vi "medicaoIXV.vi"() -> ()   [LabVIEW 2012]
uses:
  <vilib>/Utility/file.llb/Write To Spreadsheet File (string).vi
  <vilib>/Utility/file.llb/Write To Spreadsheet File (DBL).vi
  <instrlib>/Agilent 6XXX Series/Agilent 6XXX Series.lvlib
panel:
  out "PmpTemp":dbl
  out "stop2":bool
  out "reset graph":bool=TRUE
  out "array":dbl[][](array[numeric])
  in  "Tab Control":enum32{"Entrada de dados", "Saída de dados"}(tab)
  in  "Formato":u16(ring) items=[".txt", ".csv"]
  out "ON/OFF":bool
  in  "Pontos":dbl
  in  "Tensão máxima":dbl
  in  "Nome da célula":string
  in  "Local":path
  in  "Delay(ms)":dbl
  in  "Start":bool
  out "Icc (A)":dbl
  out "Vca (V)":dbl
  in  "Print Screen":bool
  out "IXV":cluster{"Y":dbl[], "Y":dbl[]}[](graph)
  out "output voltage":dbl
  out "Tensao Atual (V)":dbl
  out "Corrente Atual\n(A)":dbl
  out "Ponto Atual":i32
  out "TABELA DE DADOS\nTensão(fonte)     Tensão                  Corrente            Pontos":dbl[][](array[numeric]) caption="all rows" format="%0.3f"
  in  "stop":bool
  out "ON/OFF":bool
  in  "CorrenteGraph":dbl
  in  "error in (no error)":errorcluster
  out "error out":errorcluster
  in  "TensaoGraph":dbl
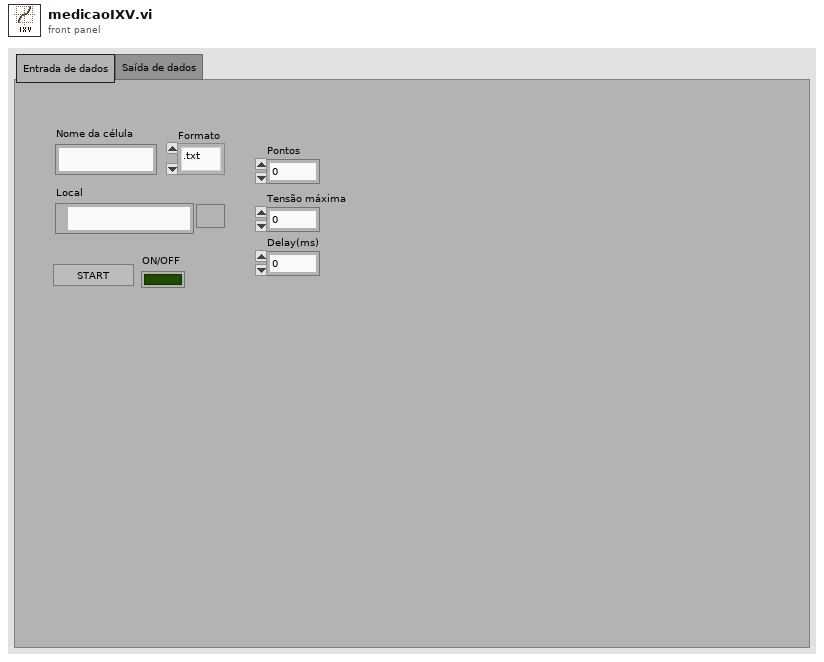
[diagram p1: front panel]
types:
  T1 = typedef "imagedata.ctl" = cluster{"image type":i32, "image depth":i32, "image":u8[], "mask":u8[], "colors":u32[], "Rectangle":cluster{"left":i16, "top":i16, "right":i16, "bottom":i16}}
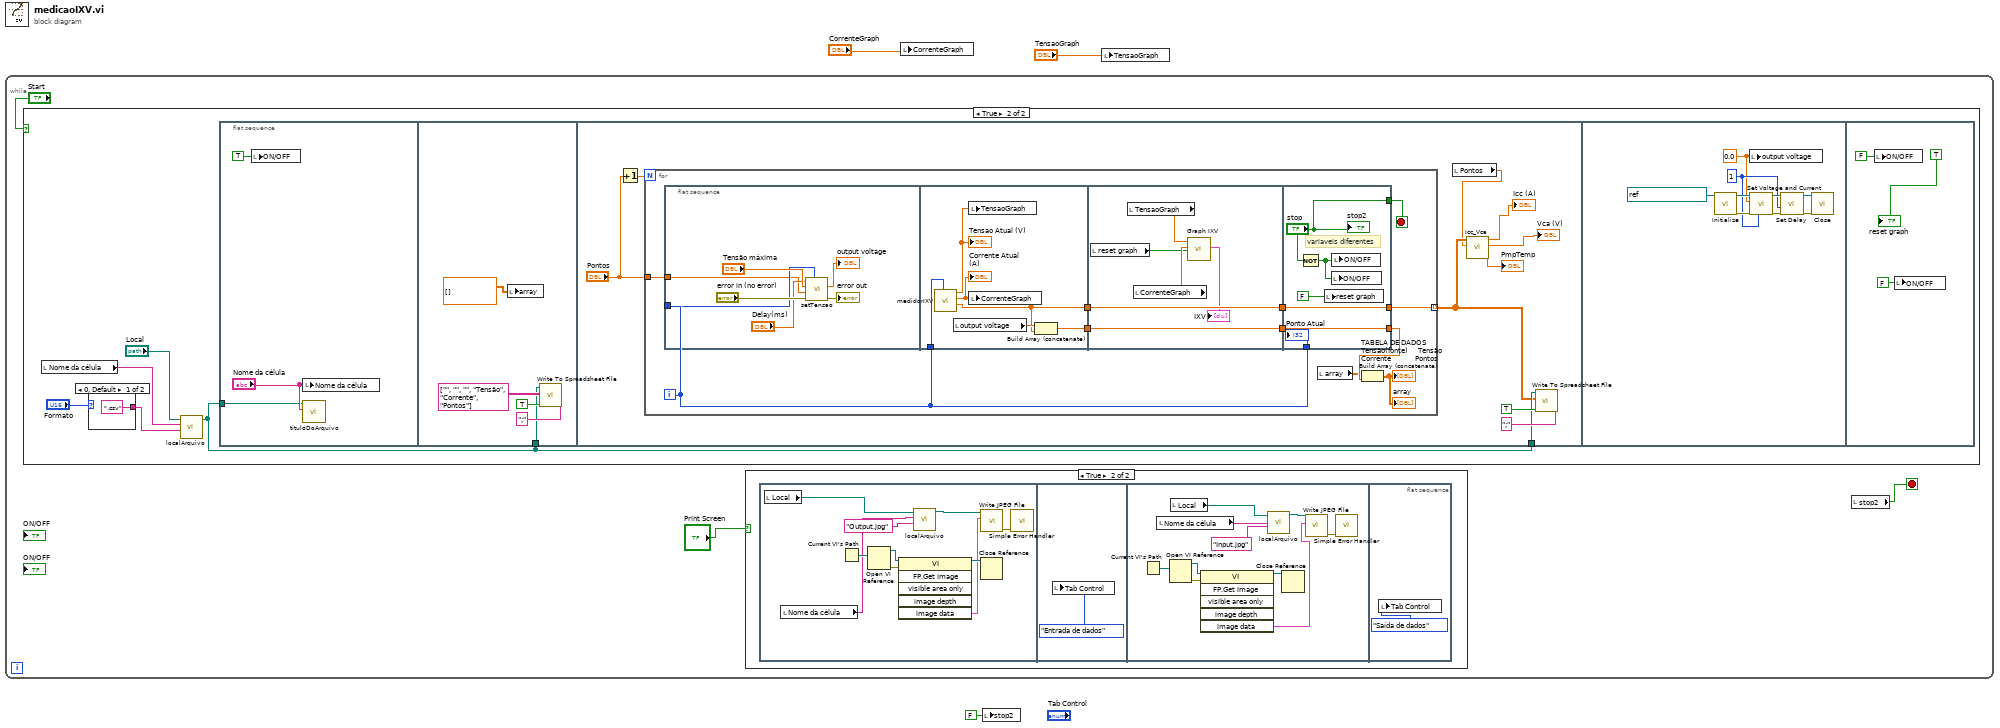
[diagram p0: block diagram]
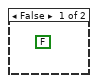
[diagram p3: hidden frame]
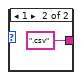
[diagram p4: hidden frame]
diagram:
  n1 = while {
    stop <- w4 stop-if-true
    n2 = case shown="True" "Start" {
      frame False {
        (unwired) FALSE
      }
      frame True {
        n3 = local read "Nome da célula"() -> (w32:string)
        n4 = case shown="0, Default" "Formato" {
          tunnel: [".csv" ".csv"] -> w29
          frame 0, Default {
          }
          frame 1 {
          }
        }
        n5 = call "localArquivo.vi"("extensão"=w29, "Nome do arquivo"=w32, "Local"="Local") -> ("Path"=w31:path)  [unwired: 8 in]
        n6 = flat-sequence {
          tunnel: w31 -> [w37]
          tunnel: w31 -> [w40]
          tunnel: w31 -> [w51]
          frame #0 {
            n7 = local write "ON/OFF"(TRUE ("ON/OFF")) -> ()
            n8 = local write "Nome da célula"("Nome da célula") -> ()
            n9 = call "tituloDoArquivo.vi"("Nome da célula"="Nome da célula", "file path (dialog if empty)"=w37) -> ()  [unwired: 10 in]
          }
          frame #1 {
            n10 = local write "array"(dbl[][] [] ("array")) -> ()
            n11 = call-poly <vilib>:"Write To Spreadsheet File.vi"("delimiter (\\t)"=";" ("delimiter (\\t)"), "append to file? (new file:F)"=TRUE, "2D data"=string[][] [["", "", ""], ["Tensão", "Corrente", "Pontos"]], "file path (dialog if empty)"=w40) -> ()  [unwired: 4 in, 1 out]
          }
          frame #2 {
            n12 = Increment(x="Pontos") -> (x+1=w50:dbl)
            n13 = for {
              N: w50 -> [_]
              tunnel: [w63] -> w47 mode=indexing
              tunnel: "Pontos" -> [w64]
              i -> [w57]
              stop <- w56 stop-if-true
              n14 = flat-sequence {
                tunnel: w64 -> [w67]
                tunnel: w57 -> [w68]
                tunnel: w57 -> [w77]
                tunnel: [w74] -> w62
                tunnel: [w76] -> w61
                tunnel: [w83] -> w55
                tunnel: [w82] -> w54
                tunnel: w61 -> [w82]
                tunnel: w62 -> [w83]
                tunnel: [w88] -> w60
                tunnel: [w89] -> w63
                tunnel: w55 -> [w89]
                tunnel: w54 -> [w88]
                tunnel: w57 -> [w87]
                tunnel: ["stop"] -> w56
                frame #0 {
                  n15 = call "setTensao.vi"("Ponto"=w68, "error in (no error)"="error in (no error)", "Pontos"=w67, "Tensão máxima"="Tensão máxima", "delay(ms)"="Delay(ms)") -> ("error out"=→"error out":errorcluster, "output voltage"=→"output voltage":dbl)  [unwired: 5 in]
                }
                frame #1 {
                  n16 = call "medidorIXV.vi"("Ponto"=w77) -> ("Array"=w74:dbl[], "Corrente Atual"=w72:dbl, "Tensao Atual"=w73:dbl)  [unwired: 8 in]
                  "Corrente Atual\n(A)" <- w72
                  "Tensao Atual (V)" <- w73
                  n17 = local read "output voltage"() -> (w75:dbl)
                  n18 = local write "TensaoGraph"(w73) -> ()
                  n19 = local write "CorrenteGraph"(w72) -> ()
                  n20 = Build Array (concatenate)(w75, w74) -> (w76:dbl[])
                }
                frame #2 {
                  n21 = local read "reset graph"() -> (w78:bool)
                  n22 = local read "TensaoGraph"() -> (w81:dbl)
                  n23 = local read "CorrenteGraph"() -> (w80:dbl)
                  n24 = call "Graph IXV"("Reset"=w78, "Y Input"=w80, "X Input"=w81) -> ("XY Graph"=→"IXV":cluster{"Y":dbl[], "Y":dbl[]}[])  [unwired: 2 in, 6 out]
                }
                frame #3 {
                  # "variaveis diferentes"
                  n25 = Not(x="stop") -> (.not. x?=w84:bool)
                  n26 = local write "reset graph"(FALSE) -> ()
                  n27 = local write "ON/OFF"(w84) -> ()
                  n28 = local write "ON/OFF"(w84) -> ()
                  "Ponto Atual" <- w87
                  "stop2" <- "stop"
                }
              }
              n29 = local read "array"() -> (w59:dbl[][])
              n30 = Build Array (concatenate)(w59, w60) -> (→"TABELA DE DADOS\nTensão(fonte)     Tensão                  Corrente            Pontos" →"array":dbl[][])
            }
            n31 = local read "Pontos"() -> (w46:dbl)
            n32 = call "Icc_Vca.vi"("VetorDeDados"=w47, "pontos"=w46) -> ("Icc"=→"Icc (A)":dbl, "Vca"=→"Vca (V)":dbl, "Pmp"=→"PmpTemp":dbl)  [unwired: 5 in]
            n33 = call-poly <vilib>:"Write To Spreadsheet File.vi"("delimiter (\\t)"=";" ("delimiter (\\t)"), "append to file? (new file:F)"=TRUE, "2D data"=w47, "file path (dialog if empty)"=w51) -> ()  [unwired: 4 in, 1 out]
          }
          frame #3 {
            w90 = 0.0 ("voltage (0 V)")
            w93 = u8 1 ("channel (1)")
            n34 = call <instrlib>:"Initialize.vi"("VISA resource name"=refnum<visa-resource-name> "GPIB0::5::INSTR") -> ("error out"=w95:errorcluster, "VISA resource name out"=w94:refnum<visa-resource-name>)  [unwired: 9 in]
            n35 = local write "output voltage"(w90) -> ()
            n36 = call <instrlib>:"Set Voltage and Current.vi"("channel (1)"=w93, "error in (no error)"=w95, "voltage (0 V)"=w90, "VISA resource name"=w94) -> ("error out"=w96:errorcluster, "VISA resource name out"=w97:refnum<visa-resource-name>)  [unwired: 6 in]
            n37 = call <instrlib>:"Set Delay.vi"("error in (no error)"=w96, "channel (1)"=w93, "VISA resource name"=w97) -> ("error out"=w91:errorcluster, "VISA resource name out"=w92:refnum<visa-resource-name>)  [unwired: 7 in]
            n38 = call <instrlib>:"Close.vi"("error in (no error)"=w91, "VISA resource name"=w92) -> ()  [unwired: 9 in, 1 out]
          }
          frame #4 {
            n39 = local write "ON/OFF"(FALSE) -> ()
            n40 = local write "ON/OFF"(FALSE ("ON/OFF")) -> ()
            "reset graph" <- TRUE
          }
        }
      }
    }
    n41 = case shown="True" "Print Screen" {
      frame False {
      }
      frame True {
        n42 = flat-sequence {
          frame #0 {
            n43 = local read "Local"() -> (w8:path)
            n44 = local read "Nome da célula"() -> (w9:string)
            n45 = Current VI's Path() -> (path=w14:path)
            n46 = Open VI Reference(vi path=w14) -> (vi reference=w15:refnum<vi>, error out=w16:errorcluster)  [unwired: 5 in]
            n47 = invoke class="VI" method="FP.Get Image"(reference=w15, error in=w16) -> (reference out=w13:refnum<vi>, "image data"=w12:T1)  [unwired: 4 in, 4 out]
            n48 = call "localArquivo.vi"("extensão"="Output.jpg", "Nome do arquivo"=w9, "Local"=w8) -> ("Path"=w7:path)  [unwired: 8 in]
            n49 = call <vilib>:"Write JPEG File.vi"("image data"=w12, "path to JPEG file"=w7) -> ("error out"=w11:errorcluster)  [unwired: 8 in, 1 out]
            n50 = Close Reference(reference=w13) -> ()  [unwired: 1 in, 1 out]
            n51 = call <vilib>:"Simple Error Handler.vi"("error in (no error)"=w11) -> ()  [unwired: 4 in, 5 out]
          }
          frame #1 {
            n52 = local write "Tab Control"(enum32{"Entrada de dados", "Saída de dados"}."Entrada de dados" ("Tab Control")) -> ()
          }
          frame #2 {
            n53 = Current VI's Path() -> (path=w26:path)
            n54 = local read "Nome da célula"() -> (w20:string)
            n55 = Open VI Reference(vi path=w26) -> (vi reference=w25:refnum<vi>, error out=w24:errorcluster)  [unwired: 5 in]
            n56 = local read "Local"() -> (w19:path)
            n57 = invoke class="VI" method="FP.Get Image"(reference=w25, error in=w24) -> (reference out=w27:refnum<vi>, "image data"=w22:T1)  [unwired: 4 in, 4 out]
            n58 = call "localArquivo.vi"("extensão"="Input.jpg", "Nome do arquivo"=w20, "Local"=w19) -> ("Path"=w18:path)  [unwired: 8 in]
            n59 = Close Reference(reference=w27) -> ()  [unwired: 1 in, 1 out]
            n60 = call <vilib>:"Write JPEG File.vi"("image data"=w22, "path to JPEG file"=w18) -> ("error out"=w23:errorcluster)  [unwired: 8 in, 1 out]
            n61 = call <vilib>:"Simple Error Handler.vi"("error in (no error)"=w23) -> ()  [unwired: 4 in, 5 out]
          }
          frame #3 {
            n62 = local write "Tab Control"(enum32{"Entrada de dados", "Saída de dados"}."Saída de dados" ("Tab Control")) -> ()
          }
        }
      }
    }
    n63 = local read "stop2"() -> (w4:bool)
  }
  n64 = local write "CorrenteGraph"("CorrenteGraph") -> ()
  n65 = local write "stop2"(FALSE ("stop2")) -> ()
  n66 = local write "TensaoGraph"("TensaoGraph") -> ()
